vi "PC_Play.vi"() -> ()   [LabVIEW 2018]
uses:
  <vilib>/Utility/file.llb/Read Delimited Spreadsheet (DBL).vi
  <resource>/objmgr/ni.dex.rc
panel:
  out "output cluster 2":T1
  out "size(s)":i32[](array[numeric])
  in  "file path (dialog if empty)":path=path "C:/Users/Silvis/Desktop/file01"
  in  "myRIO IP address":string(combo)
  out "timed out?":bool
  in  "Stop Button":bool
  out "RT reader URL":string="///RT-reader"
  out "RT connected?":bool
  # "PC host writer"
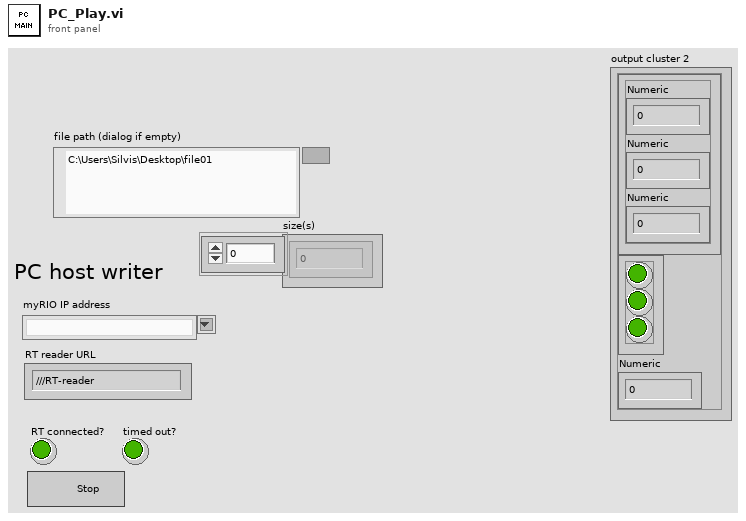
[diagram p1: front panel]
types:
  T1 = cluster{"Cluster":cluster{"Numeric":dbl, "Numeric":dbl, "Numeric":dbl}, "Cluster":cluster{"Boolean":bool, "Boolean":bool, "Boolean":bool}, "Numeric":dbl}
  T2 = cluster{"Numeric":dbl, "Numeric":dbl, "Numeric":dbl}
  T3 = cluster{cluster{"Numeric":dbl, "Numeric":dbl, "Numeric":dbl}, cluster{bool, bool, bool}, "Numeric":dbl}
  T4 = cluster{"Cluster":cluster{"Numeric":dbl, "Numeric":dbl, "Numeric":dbl}, "Cluster":cluster{"Boolean":bool, "Boolean":bool, "Boolean":bool}, "Numeric":dbl}[]
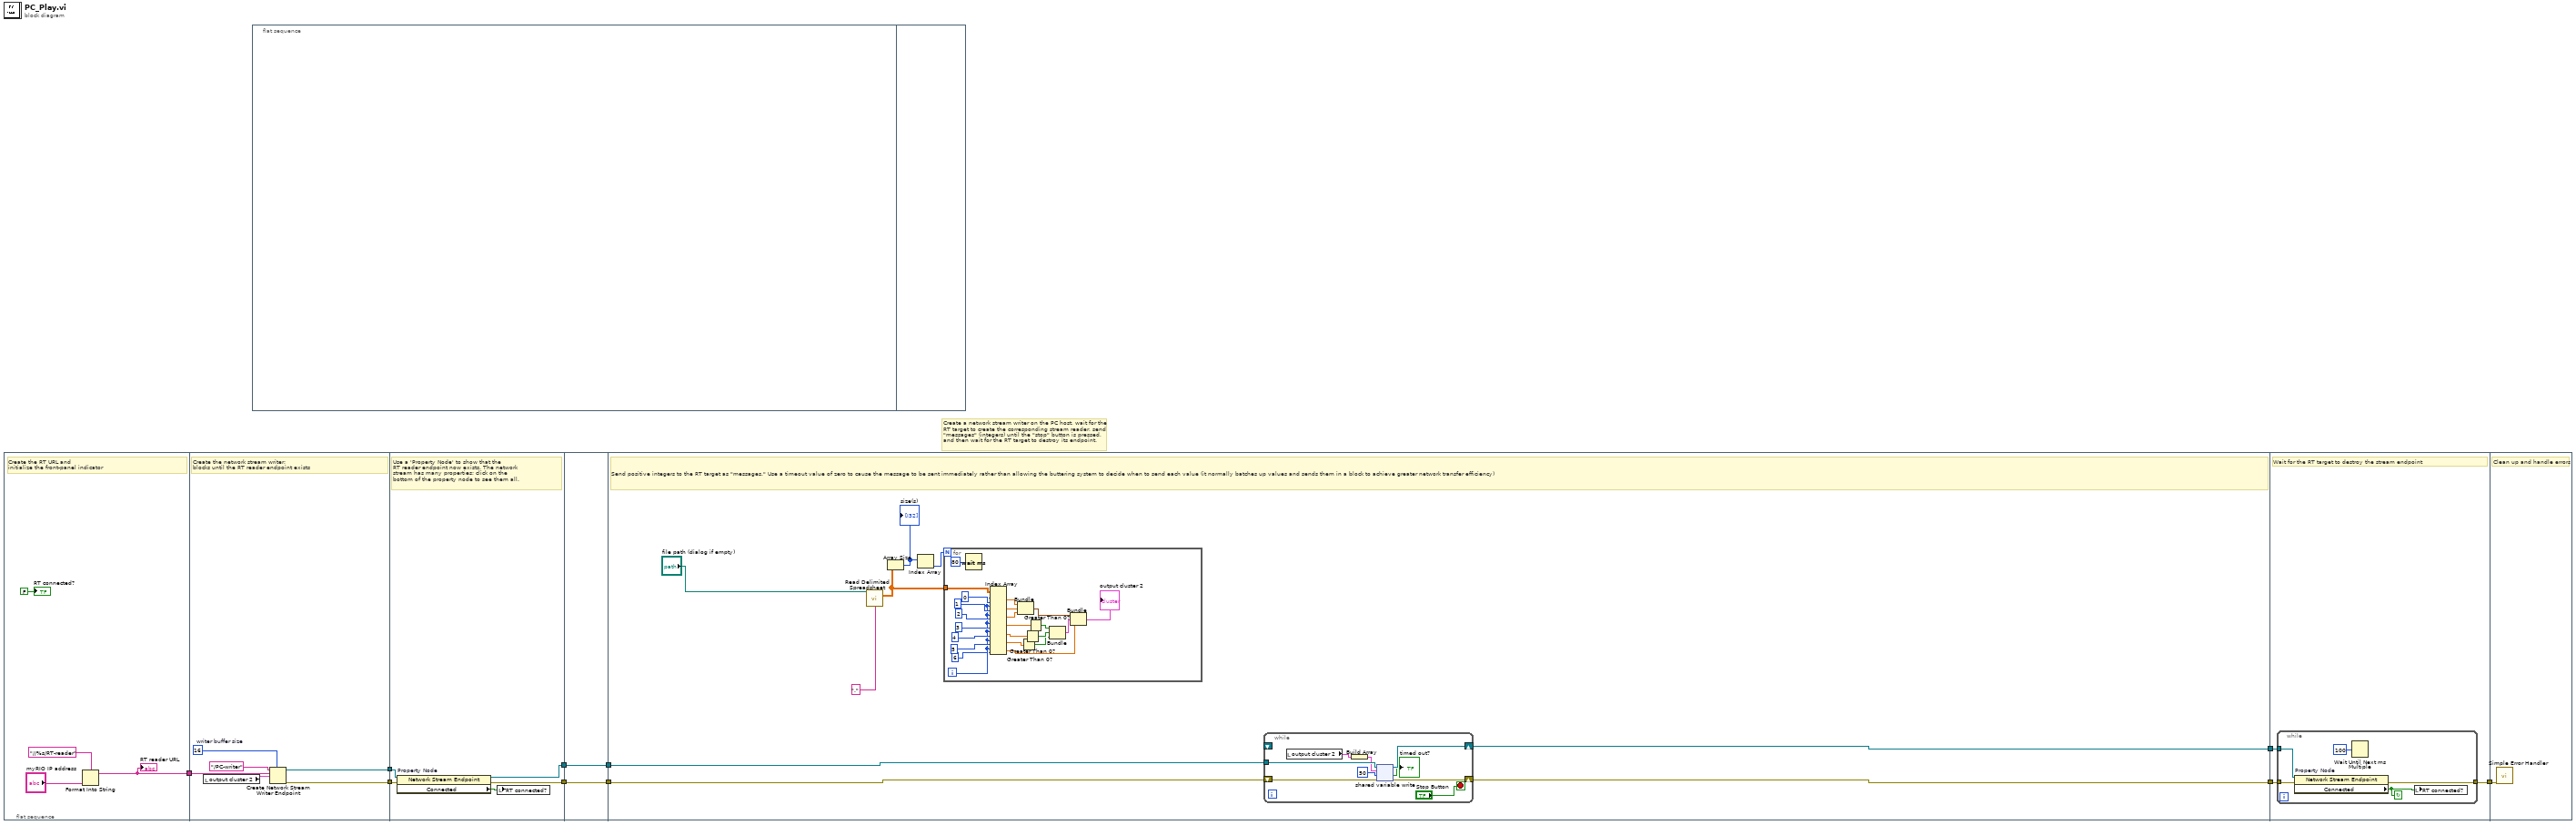
[diagram p0: block diagram]
diagram:
  # "Create a network stream writer on the PC host, wait for the\nRT target to create the corresponding stream reader, send\n\"messages\" (integers) until the \"stop\" button is pressed,\nand then wait for the RT target to destroy its endpoint."
  n1 = flat-sequence {
    tunnel: [w13] -> w10
    tunnel: w10 -> [w18]
    tunnel: [w17] -> w9
    tunnel: [w16] -> w8
    tunnel: w9 -> [w25]
    tunnel: w8 -> [w24]
    tunnel: [w23] -> w4
    tunnel: [w22] -> w2
    tunnel: w4 -> [w27]
    tunnel: [w27] -> w3
    tunnel: w2 -> [w26]
    tunnel: [w26] -> w1
    tunnel: w3 -> [w36]
    tunnel: w1 -> [w35]
    tunnel: [w34] -> w7
    tunnel: [w33] -> w6
    tunnel: w7 -> [w71]
    tunnel: w6 -> [w70]
    tunnel: [w69] -> w5
    tunnel: w5 -> [w77]
    frame #0 {
      # "Create the RT URL and\ninitialize the front-panel indicator"
      n2 = Format Into String "Format Into String"(format string="//%s/RT-reader", "myRIO IP address") -> (resulting string=w13:string)  [unwired: 2 in, 1 out]
      "RT reader URL" <- w13
      "RT connected?" <- FALSE ("RT connected?")
    }
    frame #1 {
      w20 = 16  # writer buffer size
      # "Create the network stream writer;\nblocks until the RT reader endpoint exists"
      n3 = local read "output cluster 2"() -> (w15:T1)
      n4 = Create Network Stream Writer Endpoint(7:w20, 9:w15, 10:w18, 11:"/PC-writer" ("writer name")) -> (0:w16:errorcluster, 3:w17:refnum<k21>)  [unwired: 3 in]
    }
    frame #2 {
      # "Use a 'Property Node' to show that the\nRT reader endpoint now exists. The network\nstream has many properties; click on the\nbottom of the property node to see them all."
      n5 = property on="Property Node" class="Network Stream Endpoint"(reference=w25, error in=w24) -> (reference out=w23:refnum<k21>, error out=w22:errorcluster, "Connected"=w21:bool)
      n6 = local write "RT connected?"(w21) -> ()
    }
    frame #3 {
    }
    frame #4 {
      # "Send positive integers to the RT target as \"messages.\" Use a timeout value of zero to cause the message to be sent immediately rather than allowing the buttering system to decide when to send each value (it normally batches up values and sends them in a block to achieve greater network transfer efficiency)"
      n7 = call-poly <vilib>:"Read Delimited Spreadsheet.vi"("file path (dialog if empty)"="file path (dialog if empty)", "delimiter (\\t)"="." ("delimiter (\\t)")) -> ("all rows"=w28:dbl[][])  [unwired: 8 in, 5 out]
      n8 = Array Size(array=w28) -> (size(s)=w30:i32[])
      "size(s)" <- w30
      n9 = Index Array(array=w30) -> (element=w29:i32)  [unwired: 1 in]
      n10 = for {
        N: w29 -> [_]
        tunnel: w28 -> [w58]
        i -> [w43]
        n11 = Wait (ms)(milliseconds to wait=u32 80) -> ()  [unwired: 1 out]
        n12 = Index Array(array=w58, index (row) #1=w43, index (col) #1=0 ("disabled index (row)"), index (row) #2=w43, index (col) #2=1 ("disabled index (row)"), index (row) #3=w43, index (col) #3=2 ("disabled index (row)"), index (row) #4=w43, index (col) #4=3 ("index (col)"), index (row) #5=w43, index (col) #5=4 ("index (col)"), index (row) #6=w43, index (col) #6=5 ("index (col)"), index (row) #7=w43, index (col) #7=6 ("index (col)")) -> (element #1=w57:dbl, element #2=w56:dbl, element #3=w55:dbl, element #4=w47:dbl, element #5=w42:dbl, element #6=w41:dbl, element #7=w38:dbl)
        n13 = Bundle("Numeric"=w57, "Numeric"=w56, "Numeric"=w55) -> (w54:T2)  [unwired: 1 in]
        n14 = Greater Than 0?(x=w41) -> (x > 0?=w44:bool)
        n15 = Greater Than 0?(x=w42) -> (x > 0?=w45:bool)
        n16 = Greater Than 0?(x=w47) -> (x > 0?=w46:bool)
        n17 = Bundle(w46, w45, w44) -> (w40:cluster{bool, bool, bool})  [unwired: 1 in]
        n18 = Bundle(w54, w40, "Numeric"=w38) -> (→"output cluster 2":T3)  [unwired: 1 in]
      }
      n19 = while {
        shift-right: [w64] -> w33
        shift-left: w35 -> [w65]
        tunnel: w36 -> [w67]
        shift-right: [w63] -> w34
        shift-left: _ -> [_]
        stop <- "Stop Button" stop-if-true
        n20 = local read "output cluster 2"() -> (w61:T1)
        n21 = Build Array(w61) -> (w60:T4)
        n22 = shared-variable-write(w67, w65, w60, 50 ("timeout ms (-1)")) -> (w63:refnum<k21>, w64:errorcluster, →"timed out?":bool)
      }
    }
    frame #5 {
      # "Wait for the RT target to destroy the stream endpoint"
      n23 = while {
        tunnel: w71 -> [w76]
        tunnel: w70 -> [w75]
        tunnel: [w74] -> w69
        stop <- w72 continue-if-true
        # "wait for RT to destroy the endpoint"
        n24 = property on="Property Node" class="Network Stream Endpoint"(reference=w76, error in=w75) -> (error out=w74:errorcluster, "Connected"=w72:bool)  [unwired: 1 out]
        n25 = Wait Until Next ms Multiple(millisecond multiple=u32 100) -> ()  [unwired: 1 out]
        n26 = local write "RT connected?"(w72) -> ()
      }
    }
    frame #6 {
      # "Clean up and handle errors"
      n27 = call <vilib>:"Simple Error Handler.vi"("error in (no error)"=w77) -> ()  [unwired: 4 in, 5 out]
    }
  }
  n28 = flat-sequence {
    frame #0 {
    }
    frame #1 {
    }
  }
